vi "ARRAYS TYPES.vi"() -> ()   [LabVIEW 2018]
panel:
  out "appended array":dbl[](array[numeric])
  out "output array":dbl[](array[numeric])
  out "element 3":dbl
  in  "2D ARRAY3":dbl[][](array[numeric])
  out "size(s) 5":i32[](array[numeric])
  in  "2D ARRAY 2":dbl[][](array[numeric])
  out "size(s) 4":i32[](array[numeric])
  out "element 2":dbl
  out "element":dbl
  in  "1D array 2":dbl[](array[numeric])
  out "size(s) 3":i32
  out "size(s)":i32
  in  "1D array":dbl[](array[numeric])
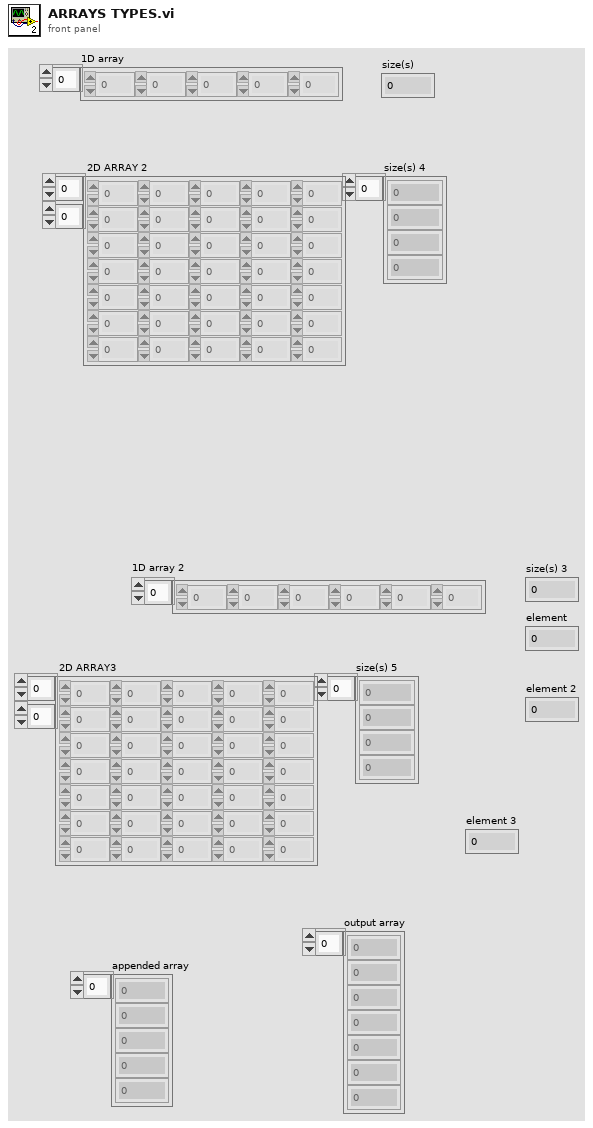
[diagram p1: front panel]
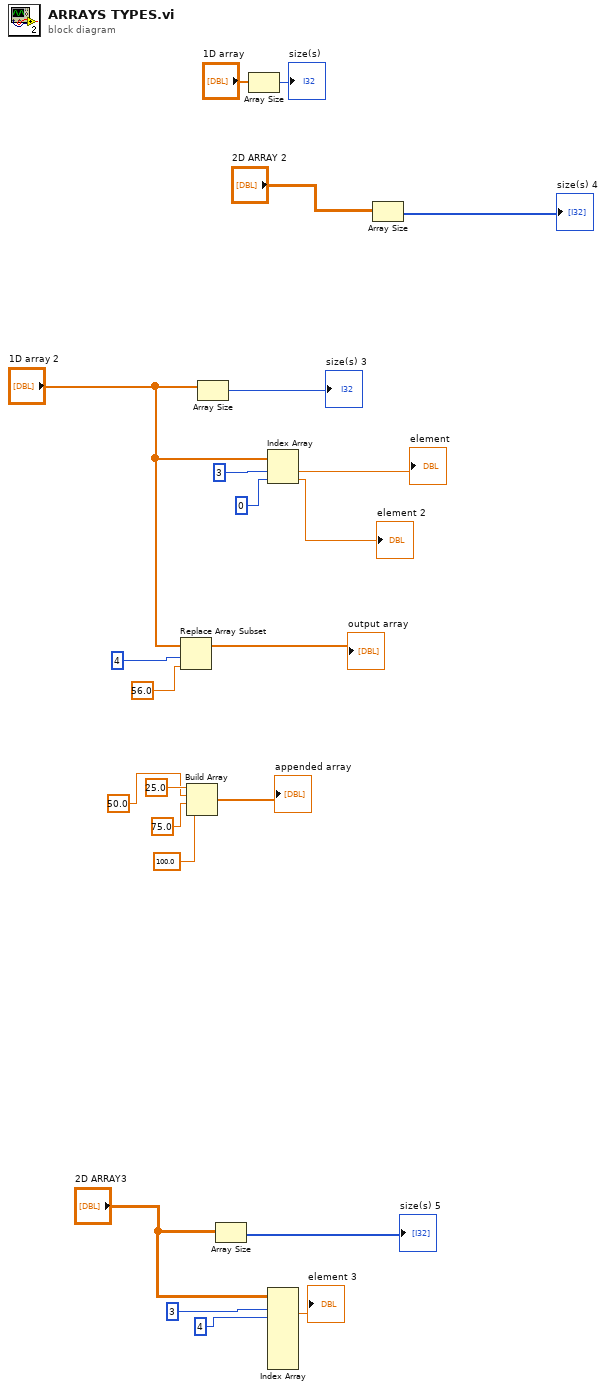
[diagram p0: block diagram]
diagram:
  n1 = Replace Array Subset "Replace Array Subset"(array="1D array 2", new element=56.0 ("new element/subarray"), index=4) -> (→"output array":dbl[])
  n2 = Build Array "Build Array"(25.0 ("element"), 50.0 ("element"), 75.0 ("element"), 100.0 ("element")) -> (→"appended array":dbl[])
  n3 = Array Size(array="1D array 2") -> (size(s)=→"size(s) 3":i32)
  n4 = Array Size(array="2D ARRAY3") -> (size(s)=→"size(s) 5":i32[])
  n5 = Array Size(array="1D array") -> (size(s)=→"size(s)":i32)
  n6 = Index Array "Index Array"(array="1D array 2", index #1=3 ("index"), index #2=0 ("index")) -> (element #1=→"element":dbl, element #2=→"element 2":dbl)
  n7 = Index Array(array="2D ARRAY3", index (row) #1=3 ("index (row)"), index (col) #1=4 ("disabled index (col)")) -> (element #1=→"element 3":dbl)  [unwired: 6 in, 3 out]
  n8 = Array Size(array="2D ARRAY 2") -> (size(s)=→"size(s) 4":i32[])
